vi "CSM MDI Example.vi"   [LabVIEW 2020]
uses:
  <userlib>/_NEVSTOP/Communicable State Machine(CSM)/_Support/GlobalEvent/GEvt-Convert Filter Rules - v1.0.vi
  b95e2d39-9a72-4fb7-b733-c53d2ceefbbe.vi
  MDI ViewManager/CSM MDI.vi
  <userlib>/_NEVSTOP/Communicable State Machine(CSM)/addons/INI-Static-Variable-Support/_Support/instances/_CSM - Read File Logger Configuration - v1.0.vi
  <userlib>/_NEVSTOP/Communicable State Machine(CSM)/addons/INI-Static-Variable-Support/_Support/instances/_CSM - Read Log Filter Rules - v1.0.vi
  <userlib>/_NEVSTOP/Communicable State Machine(CSM)/_Support/GlobalEvent/LogFilter/SettingVIs/Set Global CSM Filter.vi
  <userlib>/_NEVSTOP/Communicable State Machine(CSM)/_Support/GlobalEvent/LogFilter/SettingVIs/Set Global LogType Filter.vi
  <userlib>/_NEVSTOP/Communicable State Machine(CSM)/_Support/GlobalEvent/LogFilter/SettingVIs/Set Global State Filter.vi
  <userlib>/_NEVSTOP/Communicable State Machine(CSM)/_Support/GlobalEvent/LogFilter/SettingVIs/Set CSM LogType Filter.vi
  <userlib>/_NEVSTOP/Communicable State Machine(CSM)/_Support/GlobalEvent/LogFilter/SettingVIs/Set CSM State Filter.vi
  <userlib>/_NEVSTOP/Communicable State Machine(CSM)/_Support/GlobalEvent/LogFilter/SettingVIs/Set Global StateType Filter.vi
  <userlib>/_NEVSTOP/Communicable State Machine(CSM)/_Support/GlobalEvent/LogFilter/SettingVIs/Set CSM StateType Filter.vi
  <userlib>/_NEVSTOP/Communicable State Machine(CSM)/addons/API-String-Arugments-Support/_Support/Data To API String Arguments.vi
  <userlib>/_NEVSTOP/Communicable State Machine(CSM)/_Polymophic/Build No-Reply Asynchronous Message with Arguments.vi
  <userlib>/_NEVSTOP/Communicable State Machine(CSM)/_Support/GlobalEvent/LogFilter/LogFilter.lvclass
  <userlib>/_NEVSTOP/Communicable State Machine(CSM)/Communicable State Machine.lvlib
  MDI ViewManager/MDI ViewManager.lvlib
  <userlib>/_NEVSTOP/Communicable State Machine(CSM)/addons/INI-Static-Variable-Support/INI-Static-Variable-Support.lvlib
  <userlib>/_NEVSTOP/Communicable State Machine(CSM)/addons/Logger/CSM File Logger.lvlib
  <userlib>/_NEVSTOP/Communicable State Machine(CSM)/addons/Watchdog/CSM Watchdog.lvlib
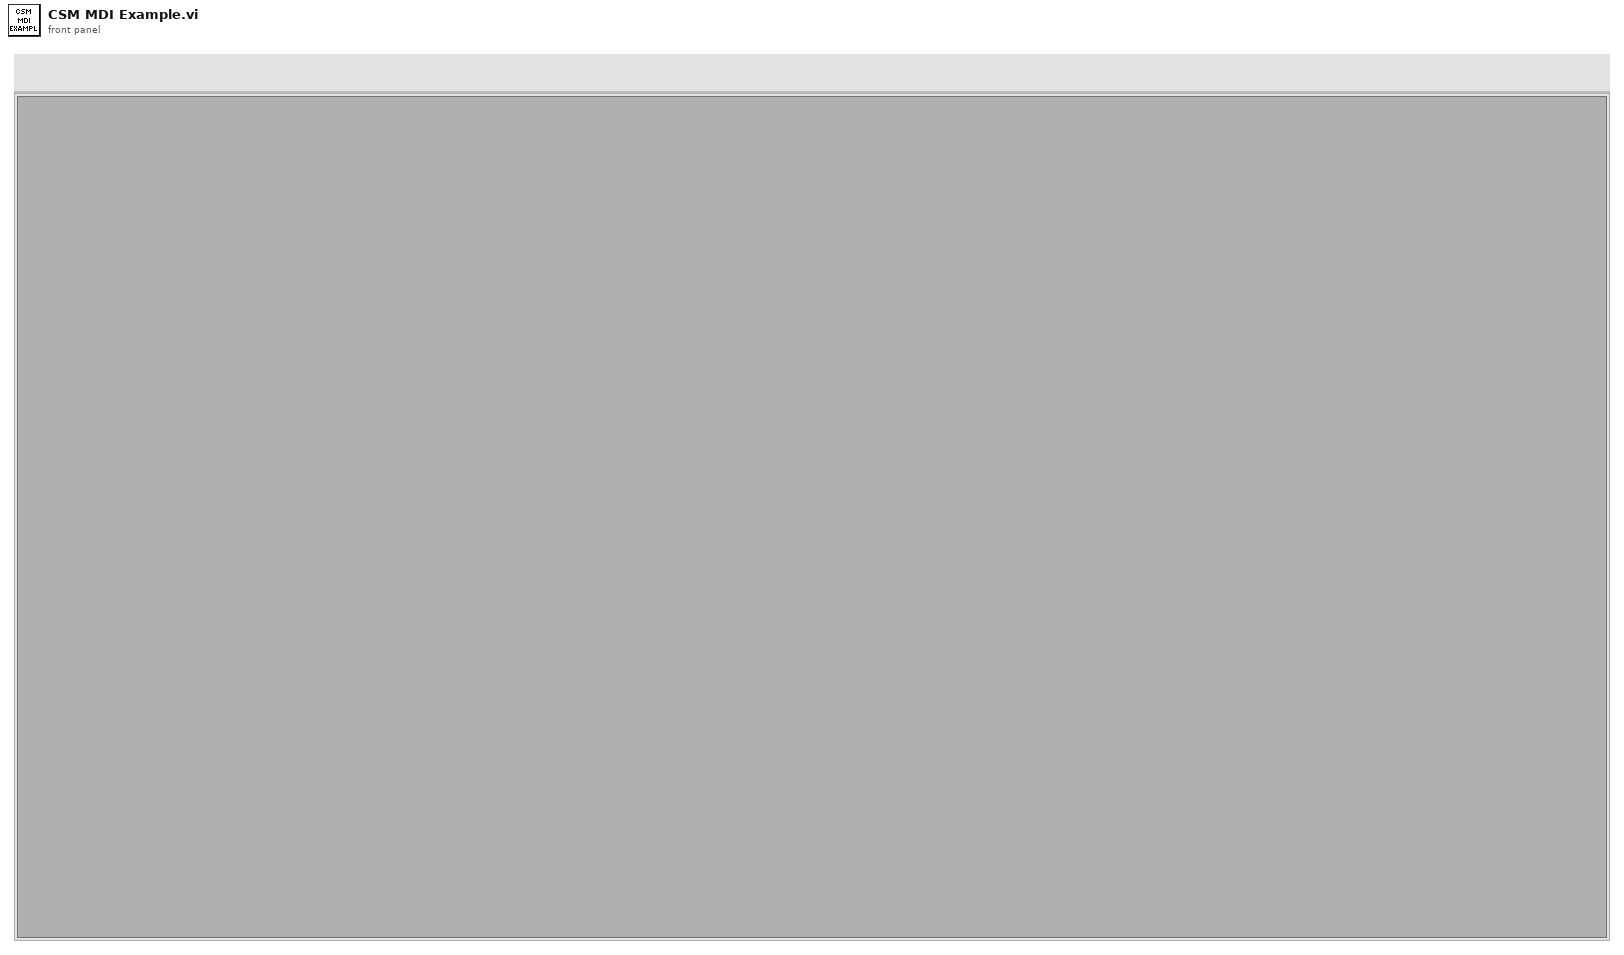
[diagram p1: front panel]
types:
  T1 = cluster{"Enable":bool, "Limit":cluster{"FileSize":i64, "FileNum":i32}, "Timestamp.Format":string, "AutoExit":bool}
  T2 = typedef "Communicable State Machine.lvlib/_CSM_GlobalLog Filter Rules - v1.0.ctl" = cluster{"Global":cluster{"CSM":string[], "LogType":T3[], "State":string[], "StateType":T4[]}, "CSM":cluster{"LogType":cluster{"CSM":string, "LogType":T3}[], "State":cluster{"CSM":string, "State":string}[], "StateType":cluster{"CSM":string, "LogType":T4}[]}}
  T3 = typedef "Communicable State Machine.lvlib/_CSM_GlobalLog_MSG_TYPE.ctl" = enum16{"User Log", "State Change", "Status", "Interrupt", "Register", "Unregister", "Error Log", "Module Created", "Module Destroyed", "Async Message", "No-Rep Async Message", "Sync Message"}
  T4 = typedef "Communicable State Machine.lvlib/_CSM_GlobalLog_STATE_TYPE.ctl" = enum16{"State - Internal State", "State - External Message", "State - Response", "State - Complete"}
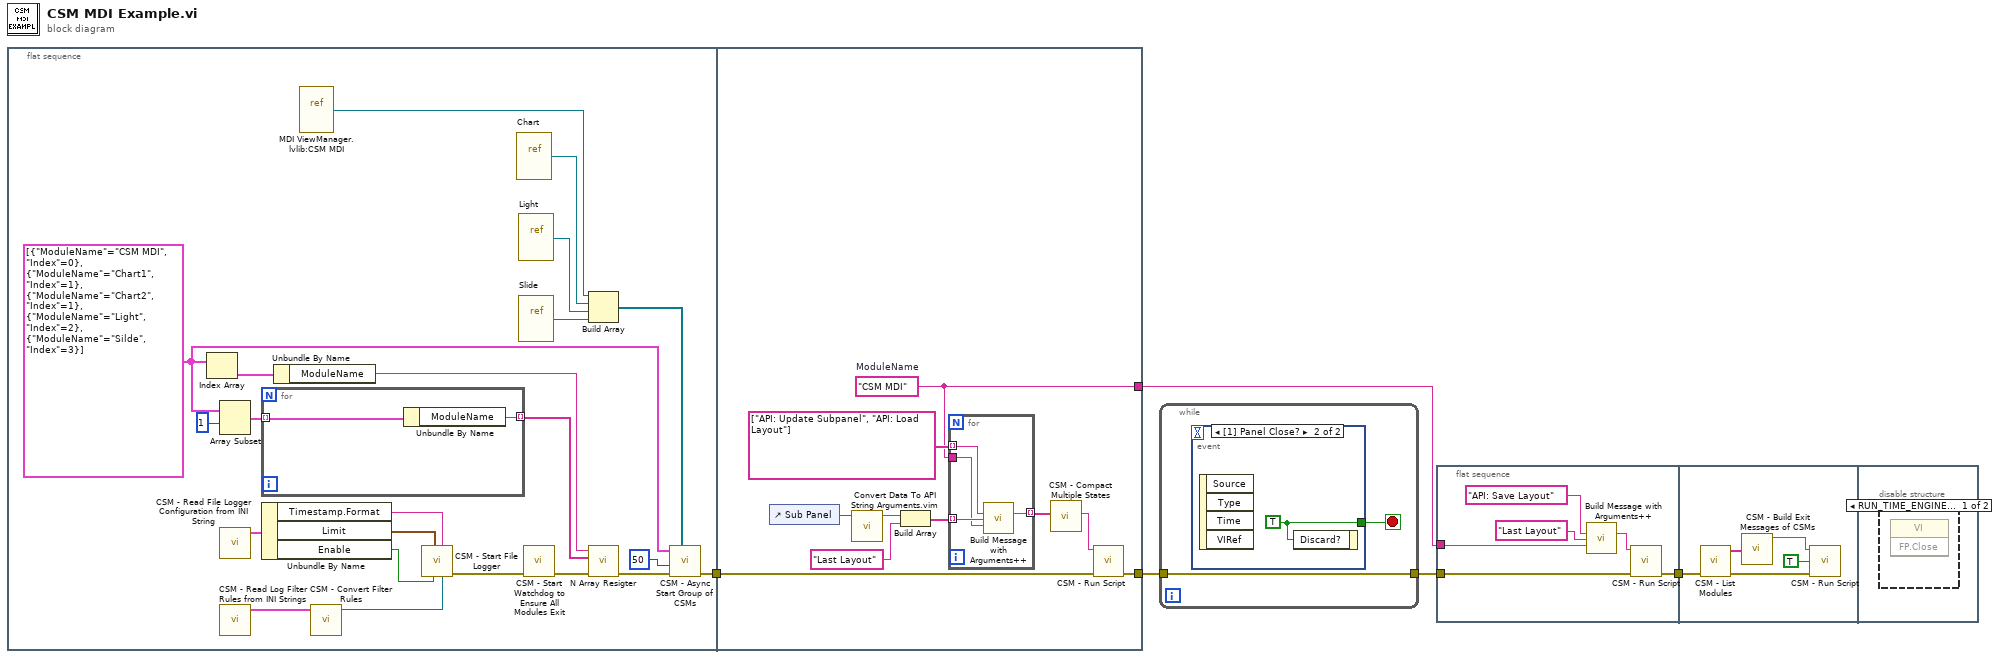
[diagram p0: block diagram]
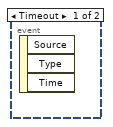
[diagram p3: hidden frame]
diagram:
  n1 = flat-sequence {
    tunnel: [w18] -> w1
    tunnel: [w30] -> w2
    tunnel: [w38] -> w3
    tunnel: w1 -> [w39]
    frame #0 {
      w20 = cluster{"ModuleName":string, "Index":i32}[] [{"ModuleName"="CSM MDI", "Index"=0}, {"ModuleName"="Chart1", "Index"=1}, {"ModuleName"="Chart2", "Index"=1}, {"ModuleName"="Light", "Index"=2}, {"ModuleName"="Silde", "Index"=3}]
      n2 = Index Array(array=w20) -> (element=w9:cluster{"ModuleName":string, "Index":i32})  [unwired: 1 in]
      n3 = Array Subset(array=w20, index=1) -> (w8:cluster{"ModuleName":string, "Index":i32}[])  [unwired: 1 in]
      n4 = call-poly <userlib>:"CSM - Read File Logger Configuration from INI String.vi"() -> ("FileLogger Configuration-v1"=w12:T1)  [unwired: 8 in, 1 out]
      n5 = call-poly <userlib>:"CSM - Read Log Filter Rules from INI Strings.vi"() -> ("Rules-v1"=w11:T2)  [unwired: 8 in, 1 out]
      n6 = for {
        tunnel: w8 -> [w29] mode=indexing
        tunnel: [w28] -> w7 mode=indexing
        n7 = Unbundle By Name(w29) -> ("ModuleName"=w28:string)
      }
      n8 = Unbundle By Name(w12) -> ("Timestamp.Format"=w15:string, "Limit"=w14:cluster{"FileSize":i64, "FileNum":i32}, "Enable"=w13:bool)
      n9 = Unbundle By Name(w9) -> ("ModuleName"=w19:string)
      n10 = vi-ref "MDI ViewManager.lvlib:CSM MDI.vi"() -> (w22:refnum<vi>)
      n11 = call-poly <userlib>:"CSM - Convert Filter Rules.vi"("Rules-v1"=w11) -> ("GlobalLogFilter"=w10:refnum<class "LogFilter.lvclass">)  [unwired: 10 in]
      n12 = call <userlib>:"CSM - Start File Logger.vi"("Filter Rules"=w10, "Timestamp Format"=w15, "Enable? (T)"=w13, "Log Limit"=w14) -> ("error out"=w16:errorcluster)  [unwired: 5 in, 2 out]
      n13 = vi-ref "Chart.vi"() -> (w26:refnum<vi>)
      n14 = vi-ref "Light.vi"() -> (w25:refnum<vi>)
      n15 = vi-ref "Slide.vi"() -> (w24:refnum<vi>)
      n16 = call <userlib>:"CSM - Start Watchdog to Ensure All Modules Exit.vi"("error in (no error)"=w16) -> ("error out"=w17:errorcluster)  [unwired: 10 in]
      n17 = Build Array(w22, w26, w25, w24) -> (w23:refnum<vi>[])
      n18 = call "N Array Resigter.vi"("error in (no error)"=w17, "Event Source"=w7, "Taget"=w19) -> ("error out"=w21:errorcluster)  [unwired: 8 in]
      n19 = call "CSM - Async Start Group of CSMs.vi"("Prototypes"=w23, "error in (no error)"=w21, "interval(50ms)"=u32 50, "Module List"=w20) -> ("error out"=w18:errorcluster)  [unwired: 5 in]
    }
    frame #1 {
      w30 = "CSM MDI"  # ModuleName
      n20 = control-ref of="Sub Panel"() -> (w33:refnum<vi>)
      n21 = call "Convert Data To API String Arguments.vim"("Data"=w33) -> ("API String"=w34:string)  [unwired: 7 in, 1 out]
      n22 = Build Array(w34, "Last Layout" ("State With Arguments")) -> (w32:string[])
      n23 = for {
        tunnel: string[] ["API: Update Subpanel", "API: Load Layout"] ("State With Arguments") -> [w43] mode=indexing
        tunnel: w32 -> [w42] mode=indexing
        tunnel: [w41] -> w37 mode=indexing
        tunnel: w30 -> [w40]
        n24 = call-poly <userlib>:"Build Message with Arguments++.vi"("State With Arguments"=w43, "Arguments (\"\")"=w42, "Target Module (\"\")"=w40) -> ("CSM Message String"=w41:string)  [unwired: 12 in]
      }
      n25 = call <userlib>:"CSM - Compact Multiple States.vi"("Multiple States"=w37) -> ("States"=w35:string)  [unwired: 9 in]
      n26 = call <userlib>:"CSM - Run Script.vi"("CSM Scripts"=w35, "error in (no error)"=w39) -> ("error out"=w38:errorcluster)  [unwired: 11 in, 2 out]
    }
  }
  n27 = while {
    tunnel: w3 -> [w44]
    tunnel: [w44] -> w5
    stop <- w45 stop-if-true
    n28 = event shown="[1] Panel Close?" {
      selector: _ -> [_ _]
      dyn-events: _ -> [_ _]
      timeout: _ -> [_ _]
      tunnel: [_ w46] -> w45
      event Timeout {
        n29 = event-data() -> ()  [unwired: 1 in, 3 out]
      }
      event Panel Close? {
        w46 = TRUE ("Discard?")
        n30 = event-data() -> ()  [unwired: 1 in, 4 out]
        n31 = event-data("Discard?"=w46) -> ()  [unwired: 1 in, 1 out]
      }
    }
  }
  n32 = flat-sequence {
    tunnel: w5 -> [w50]
    tunnel: [w49] -> w4
    tunnel: w2 -> [w48]
    tunnel: w4 -> [w54]
    frame #0 {
      n33 = call-poly <userlib>:"Build Message with Arguments++.vi"("State With Arguments"="API: Save Layout", "Arguments (\"\")"="Last Layout" ("State With Arguments"), "Target Module (\"\")"=w48) -> ("CSM Message String"=w51:string)  [unwired: 12 in]
      n34 = call <userlib>:"CSM - Run Script.vi"("CSM Scripts"=w51, "error in (no error)"=w50) -> ("error out"=w49:errorcluster)  [unwired: 11 in, 2 out]
    }
    frame #1 {
      # "关闭所有CSM模块"
      n35 = call <userlib>:"CSM - List Modules.vi"("Error In"=w54) -> ("error out"=w53:errorcluster, "Module Names"=w55:string[])  [unwired: 9 in]
      n36 = call <userlib>:"CSM - Build Exit Messages of CSMs.vi"("CSMs"=w55) -> ("States"=w57:string)  [unwired: 14 in]
      n37 = call <userlib>:"CSM - Run Script.vi"("CSM Scripts"=w57, "Continue If Error? (F)"=TRUE, "error in (no error)"=w53) -> ()  [unwired: 10 in, 3 out]
    }
    frame #2 {
      n38 = disable-structure shown="RUN_TIME_ENGINE==True" {
        frame condition #0 {
          n39 = invoke class="VI" method="FP.Close"() -> ()  [unwired: 3 in, 3 out]
        }
        frame condition #1 (active) {
        }
      }
    }
  }
